vi "AIT 1553 - RT Driver Init.vi"(0 "Device Reference in":T1 format="%.0x", 11 "error in":errorcluster) -> (4 "Device Reference out":T1 format="%.0x", 6 "1553 Hardware Type":T3, 8 "Bus Config Info":T2, 10 "Bus Config Info Array":T2[](array[typedef]), 14 "Child Refs - 1553 Busses":T1[](array[typedef]) format="%.0x", 15 "error out":errorcluster)   [LabVIEW 2015, in "AIT 1553 Custom Device.lvlib"]
uses:
  AIT 1553 Custom Device.lvlib
  <vilib>/NI Veristand/Custom Device API/Custom Device Item Ref.ctl
  RT Controls/AIT 1553 - Hardware Type.ctl
  RT Controls/AIT 1553 - Board Config Info.ctl
  <vilib>/NI Veristand/Custom Device Tools/Custom Device Utility Library/RT Debug String Color Spec.ctl
  <vilib>/NI Veristand/Custom Device API/Get Item Property (Variant).vi
  <vilib>/NI Veristand/Custom Device API/Get Item Property (Path).vi
  <vilib>/NI Veristand/Custom Device API/Get Item Property (U32).vi
  Controls and Global/Global.vi
  <instrlib>/AIT 1553/Private/AIT 1553 Initialize/AIT 1553 Initialize (Index).vi
  <vilib>/NI Veristand/Custom Device API/Get Item Property (U16).vi
  <vilib>/NI Veristand/Custom Device API/Custom Device API.lvlib
  <instrlib>/AIT 1553/AIT 1553.lvlib
  <userlib>/MIL-STD-1553/Owl1553.lvlib
  <vilib>/NI Veristand/Custom Device Tools/Custom Device Utility Library/Custom Device Utility Library.lvlib
panel:
  out "board":T4
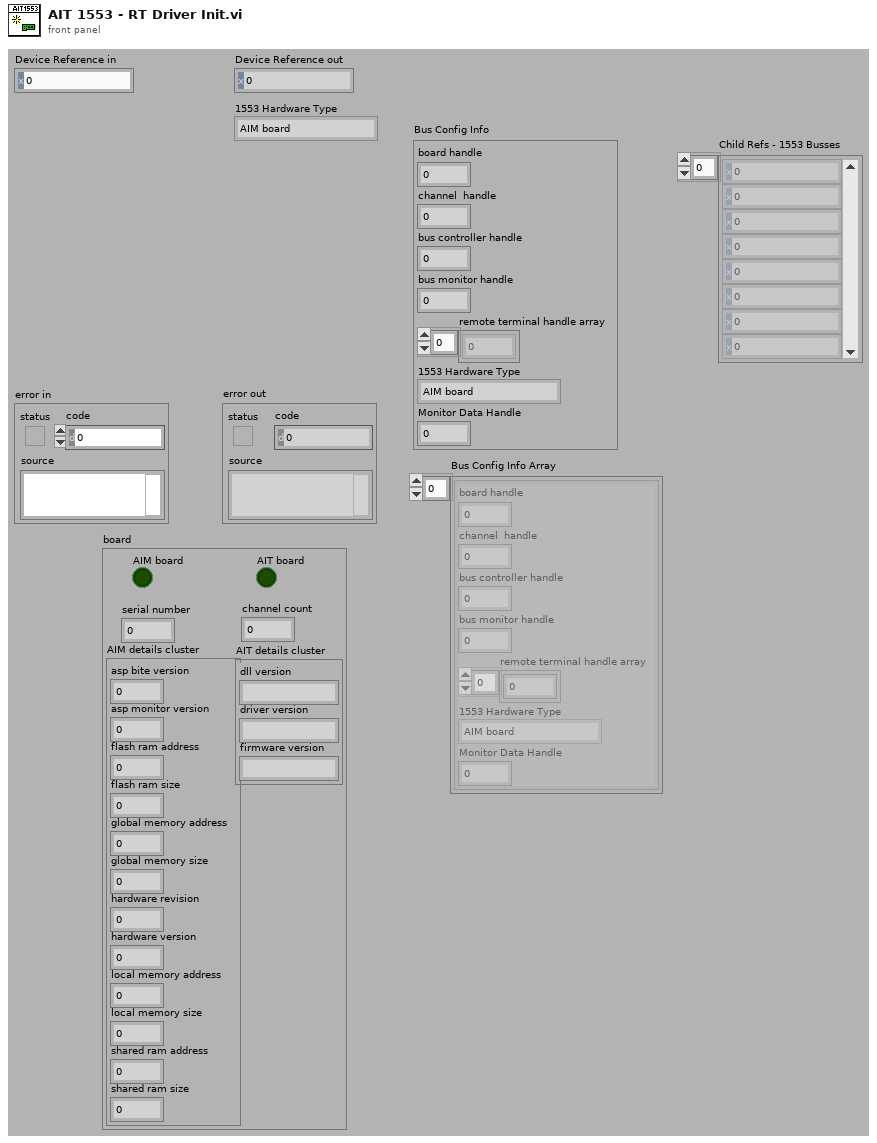
[diagram p1: front panel]
types:
  T1 = typedef "Custom Device API.lvlib/Custom Device Item Ref.ctl" = u64
  T2 = typedef "AIT 1553 Custom Device.lvlib/AIT 1553 - Board Config Info.ctl" = cluster{"board handle":u32, "channel  handle":u32, "bus controller handle":u32, "bus monitor handle":u32, "remote terminal handle array":u32[], "1553 Hardware Type":T3, "Monitor Data Handle":u32}
  T3 = typedef "AIT 1553 Custom Device.lvlib/AIT 1553 - Hardware Type.ctl" = enum16{"AIM board", "AIT Board"}
  T4 = cluster{"AIM board":bool, "AIT board":bool, "serial number":u64, "channel count":u8, "AIM details cluster":cluster{"asp bite version":u32, "asp monitor version":u32, "flash ram address":u32, "flash ram size":u32, "global memory address":u32, "global memory size":u32, "hardware revision":u32, "hardware version":u32, "local memory address":u32, "local memory size":u32, "shared ram address":u32, "shared ram size":u32}, "AIT details cluster":cluster{"dll version":string, "driver version":string, "firmware version":string}}
  T5 = typedef "Custom Device Utility Library.lvlib/RT Debug String Color Spec.ctl" = u16
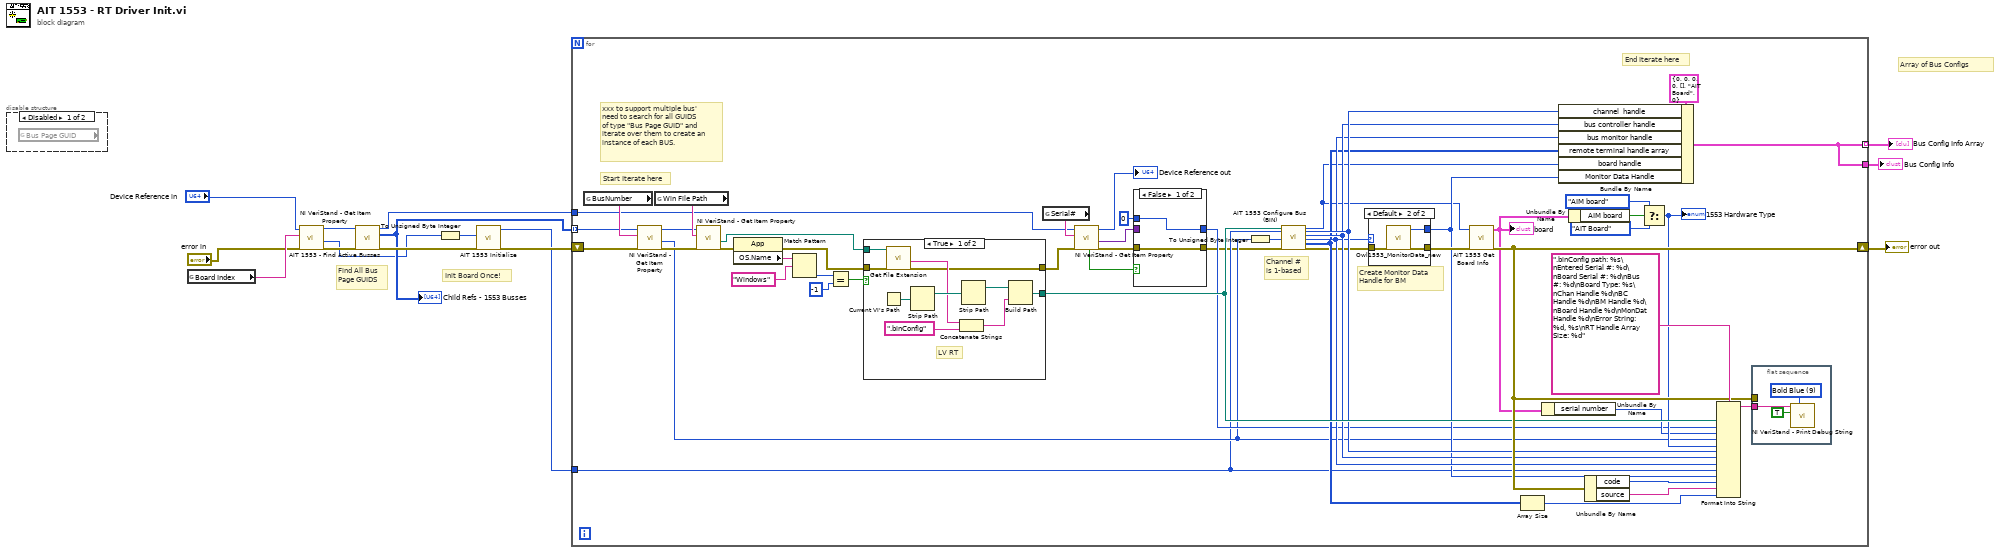
[diagram p0: block diagram]
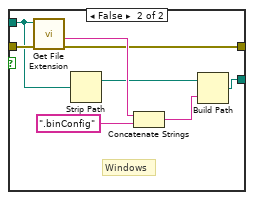
[diagram p4: hidden frame]
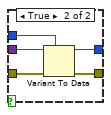
[diagram p5: hidden frame]
diagram:
  # "Find All Bus\nPage GUIDS"
  # "Init Board Once!"
  # "Array of Bus Configs"
  n1 = disable-structure shown="Disabled" {
    frame Disabled {
      n2 = global read "Global.vi" "Bus Page GUID"() -> ()  [unwired: 1 out]
    }
    frame Enabled {
    }
  }
  n3 = global read "Global.vi" "Board Index"() -> (w8:string)
  n4 = call-poly <vilib>:"NI VeriStand - Get Item Property.vi"("error in (no error)"="error in", "Property Name"=w8, "Item Ref in"="Device Reference in") -> ("error out"=w9:errorcluster, "Value"=w6:u16, "Item Ref out"=w7:T1)  [unwired: 5 in, 1 out]
  n5 = call "AIT 1553 - Find Active Busses.vi"("Device Item Ref in"=w7, "error in (no error)"=w9) -> ("Device Item Ref out"=w12:T1, "Child Refs - 1553 Busses"=w11:T1[], "error out"=w14:errorcluster)  [unwired: 11 in]
  "Child Refs - 1553 Busses" <- w11
  n6 = To Unsigned Byte Integer(number=w6) -> (unsigned 8bit integer=w5:u8)
  n7 = call-poly <instrlib>:"AIT 1553 Initialize.vi"("error in"=w14, "board index in"=w5) -> ("error out"=w13:errorcluster, "board handle out"=w10:u64)  [unwired: 8 in]
  n8 = for {
    tunnel: [w16] -> w4 mode=indexing
    tunnel: w12 -> [w23]
    tunnel: w11 -> [w22] mode=indexing
    tunnel: w10 -> [w21]
    shift-right: [w44] -> w15
    shift-left: w13 -> [w24]
    tunnel: [w16] -> w3
    # "Channel #\nis 1-based"
    # "End Iterate here"
    # "Start Iterate here"
    # "xxx to support multiple bus'\nneed to search for all GUIDS\nof type \"Bus Page GUID\" and\niterate over them to create an\ninstance of each BUS."
    # "Create Monitor Data\nHandle for BM"
    n9 = global read "Global.vi" "BusNumber"() -> (w28:string)
    n10 = call-poly <vilib>:"NI VeriStand - Get Item Property.vi"("error in (no error)"=w24, "Property Name"=w28, "Item Ref in"=w22) -> ("error out"=w30:errorcluster, "Value"=w25:u32, "Item Ref out"=w29:T1)  [unwired: 5 in, 1 out]
    n11 = global read "Global.vi" "Win File Path"() -> (w31:string)
    n12 = call-poly <vilib>:"NI VeriStand - Get Item Property.vi"("error in (no error)"=w30, "Property Name"=w31, "Item Ref in"=w29) -> ("error out"=w60:errorcluster, "Value"=w55:path)  [unwired: 5 in, 2 out]
    n13 = property class="App"(error in=w60) -> (error out=w56:errorcluster, "OS.Name"=w52:string)  [unwired: 1 in, 1 out]
    n14 = Match Pattern(string=w52, regular expression="Windows") -> (offset past match=w58:i32)  [unwired: 1 in, 3 out]
    n15 = Equal?(x=w58, y=-1) -> (x = y?=w53:bool)
    n16 = case shown="True" w53 {
      tunnel: w56 -> [w73 w85]
      tunnel: w55 -> [w76 w84]
      tunnel: [w75 w87] -> w54
      tunnel: [w74 w86] -> w42
      frame True {
        # "LV RT"
        n17 = Current VI's Path() -> (path=w78:path)
        n18 = call <vilib>:"Get File Extension.vi"("error in (no error)"=w73, "file"=w76) -> ("error out"=w75:errorcluster, "filename without extension"=w77:string)  [unwired: 5 in, 3 out]
        n19 = Strip Path(path=w78) -> (stripped path=w79:path)  [unwired: 1 out]
        n20 = Concatenate Strings(w77, ".binConfig" ("string")) -> (w81:string)
        n21 = Strip Path(path=w79) -> (stripped path=w80:path)  [unwired: 1 out]
        n22 = Build Path(base path=w80, name or relative path=w81) -> (appended path=w74:path)
      }
      frame False {
        # "Windows"
        n23 = call <vilib>:"Get File Extension.vi"("error in (no error)"=w85, "file"=w84) -> ("error out"=w87:errorcluster, "filename without extension"=w88:string)  [unwired: 5 in, 3 out]
        n24 = Strip Path(path=w84) -> (stripped path=w83:path)  [unwired: 1 out]
        n25 = Concatenate Strings(w88, ".binConfig" ("string")) -> (w89:string)
        n26 = Build Path(base path=w83, name or relative path=w89) -> (appended path=w86:path)
      }
    }
    n27 = global read "Global.vi" "Serial#"() -> (w65:string)
    n28 = call-poly <vilib>:"NI VeriStand - Get Item Property.vi"("error in (no error)"=w54, "Property Name"=w65, "Item Ref in"=w23) -> ("error out"=w64:errorcluster, "Value"=w62:variant, "Item Ref out"=→"Device Reference out":T1, "Found?"=w63:bool)  [unwired: 5 in]
    n29 = case shown="False" w63 {
      tunnel: w64 -> [w92 w97]
      tunnel: w62 -> [_ w96]
      tunnel: u64 0 -> [w91 w95]
      tunnel: [w92 w94] -> w20
      tunnel: [w91 w93] -> w26
      frame False {
      }
      frame True {
        n30 = Variant To Data(error in=w97, type=w95, Variant=w96) -> (data=w93:u64, error out=w94:errorcluster)
      }
    }
    n31 = To Unsigned Byte Integer(number=w25) -> (unsigned 8bit integer=w19:u8)
    n32 = call <instrlib>:"AIT 1553 Configure Bus (BIN).vi"("Binary File path"=w42, "board handle"=w21, "channel number"=w19, "error in"=w20) -> ("board handle"=w17:u64, "channel  handle"=w39:u64, "bus controller handle"=w38:u64, "bus monitor handle"=w37:u64, "remote terminal handle array"=w35:u64[], "error out"=w18:errorcluster)  [unwired: 10 in]
    n33 = case shown="Default" w37 {
      tunnel: w18 -> [w66 w69]
      tunnel: [w66 w68] -> w43
      tunnel: [_ w67] -> w36
      frame 0 {
      }
      frame Default {
        n34 = call <userlib>:"Owl1553_MonitorData_new.vi"("error in (no error)"=w69) -> ("error out"=w68:errorcluster, "monitor data handle"=w67:u64)  [unwired: 9 in]
      }
    }
    n35 = call <instrlib>:"AIT 1553 Get Board Info.vi"("error in"=w43, "board handle in"=w17) -> ("error out"=w44:errorcluster, "board"=w33:T4)  [unwired: 8 in]
    "board" <- w33
    n36 = Array Size(array=w35) -> (size(s)=w34:i32)
    n37 = Unbundle By Name(w33) -> ("serial number"=w27:u64)
    n38 = Bundle By Name(cluster=T2 {"board handle"=0, "channel  handle"=0, "bus controller handle"=0, "bus monitor handle"=0, "remote terminal handle array"=[], "1553 Hardware Type"=enum."AIT Board", "Monitor Data Handle"=0} ("Bus Config Info"), "channel  handle"=w39, "bus controller handle"=w38, "bus monitor handle"=w37, "remote terminal handle array"=w35, "board handle"=w17, "Monitor Data Handle"=w36) -> (w16:T2)
    n39 = Unbundle By Name(w33) -> ("AIM board"=w50:bool)
    n40 = Unbundle By Name(w44) -> ("code"=w40:i32, "source"=w41:string)
    n41 = Select(t=AIT_1553_-_Hardware_Type."AIM board" ("1553 Hardware Type"), s=w50, f=AIT_1553_-_Hardware_Type."AIT Board" ("1553 Hardware Type")) -> (s? t:f=w32:T3)
    "1553 Hardware Type" <- w32
    n42 = Format Into String(format string=".binConfig path: %s\nEntered Serial #: %d\nBoard Serial #: %d\nBus #: %d\nBoard Type: %s\nChan Handle %d\nBC Handle %d\nBM Handle %d\nBoard Handle %d\nMonDat Handle %d\nError String: %d, %s\nRT Handle Array Size: %d", w42, w26, w27, w25, w32, w39, w38, w37, w21, w36, w40, w41, w34) -> (resulting string=w45:string)  [unwired: 2 in, 1 out]
    n43 = flat-sequence {
      tunnel: w45 -> [w72]
      tunnel: w44 -> [_]
      frame #0 {
        w71 = T5 9 items=["Plain White"=7, "Bold White"=15, "Bold Blue"=9, "Bold Green"=10, "Bold Red"=12] ("Attribute")
        n44 = call <vilib>:"NI VeriStand - Print Debug String.vi"("Attribute"=w71, "Add to log file? (T)"=TRUE, "Message"=w72) -> ()  [unwired: 8 in, 1 out]
      }
    }
  }
  "error out" <- w15
  "Bus Config Info" <- w3
  "Bus Config Info Array" <- w4
